vi "Lockin.Low Pass Filter Bank 2D DO NOT USE.vi"(8 "error in (no error)":errorcluster, 10 "WFms in":waveform(dbl)[][](array[waveform]), 11 "Instrument.DAQ in":refnum<class "Instrument.DAQ.lvclass">) -> (0 "error out":errorcluster, 2 "Wfms out":waveform(dbl)[][](array[waveform]), 3 "Instrument.DAQ out":refnum<class "Instrument.DAQ.lvclass">)   [LabVIEW 2019, in "Instrument.Lockin.lvlib" / "Instrument.DAQ.lvclass"]
uses:
  Instrument.DAQ.lvclass
  <vilib>/addons/Digital Filter Design/NI_DigFilterLicensed.lvlib
  <vilib>/addons/Digital Filter Design/Process.llb/DFD Filtering with State (Wfm).vi
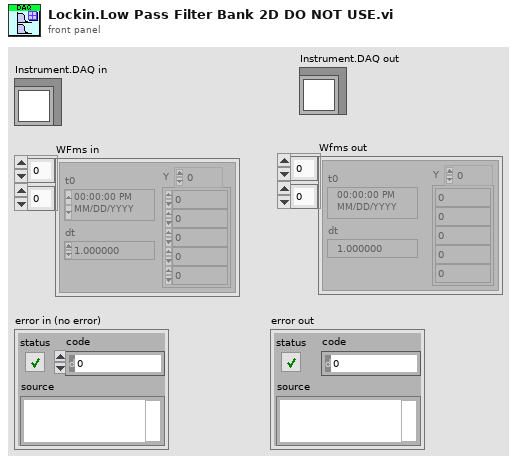
[diagram p1: front panel]
types:
  T1 = enum16{"Lowpass", "Highpass", "Bandpass", "Bandstop"}
  T2 = typedef "NI_DigFilterLicensed.lvlib/DFD Filter Obj.ctl" = cluster{"mSRate_Fs":dbl, "mSRate_Version":string, "mSRate_Comments":string, "mSRate_OrgCoef":T3, "mSRate_CurCoef":T3, "mSRate_Quantized?":bool, "mSRate_QCoef":T3, "mSRate_QSettings":T5[], "mSRate_Order":i32, "mSRate_Scaling":cluster{"mSRate_ScaleByPowerOf2?":bool, "mSRate_ScaleType":T7}}
  T3 = typedef "NI_DigFilterLicensed.lvlib/DFD Filter Coef.ctl" = cluster{"type":T4, "gain":dbl, "coef a (k)":dbl[], "coef b (v)":dbl[]}
  T4 = typedef "NI_DigFilterLicensed.lvlib/DFD Filter Structure Type Selector.ctl" = enum16{"Undefined", "FIR Direct Form", "FIR Direct Form Transposed", "FIR Symmetric", "FIR Antisymmetric", "IIR Direct Form I", "IIR Direct Form I Transposed", "IIR Direct Form II", "IIR Direct Form II Transposed", "IIR Cascaded Second Order Sections Form I", "IIR Cascaded Second Order Sections Form I Transposed", "IIR Cascaded Second Order Sections Form II", "IIR Cascaded Second Order Sections Form II Transposed", "Lattice Allpass (basic sections)", "Lattice Allpass (one multiplier sections)", "Lattice Allpass (normalized sections)", "Lattice AR (basic sections)", "Lattice AR (one multiplier sections)", "Lattice AR (normalized sections)", "Lattice MA (minimum phase)", "Lattice MA (maximum phase)", "Lattice ARMA (basic sections)", "Lattice ARMA (one multiplier sections)", "Lattice ARMA (normalized sections)"}
  T5 = typedef "NI_DigFilterLicensed.lvlib/dfd_Internal Quantization Settings.ctl" = cluster{"source":T6, "wl":i16, "iwl":i16, "overflow mode":enum16{"Saturation", "Wrap"}, "rounding mode":enum16{"Nearest", "Truncation"}, "signed?":bool}
  T6 = typedef "NI_DigFilterLicensed.lvlib/dfd_Internal Quantization Srcs.ctl" = u16
  T7 = typedef "NI_DigFilterLicensed.lvlib/DFD Coef Norm Type.ctl" = enum16{"No Norm", "Time Domain 1-Norm", "Time Domain 2-Norm", "Time Domain Inf-Norm"}
  T8 = typedef "Instrument.Lockin.lvlib/Instrument.DAQ.lvclass/REF.Channel--Cluster--Array.ctl" = T9[]
  T9 = typedef "Instrument.Lockin.lvlib/Instrument.DAQ.lvclass/REF.Channel--Cluster.ctl" = cluster{"Enable?":bool, "Channel":i32, "Frequency":dbl, "Phase":dbl, "TC":dbl, "Roll-Off":i32}
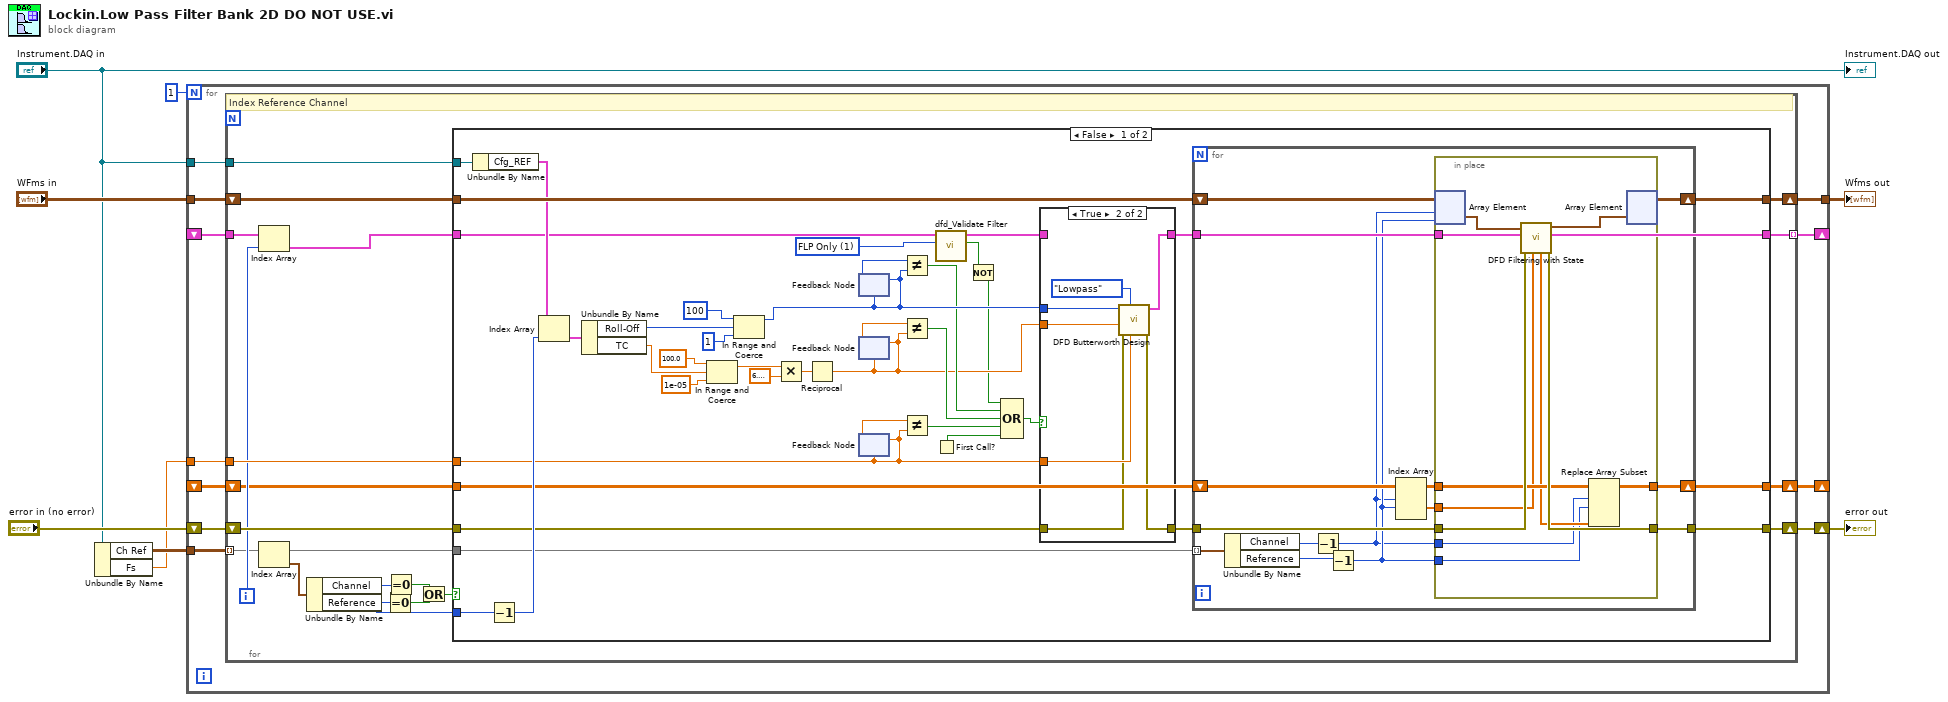
[diagram p0: block diagram]
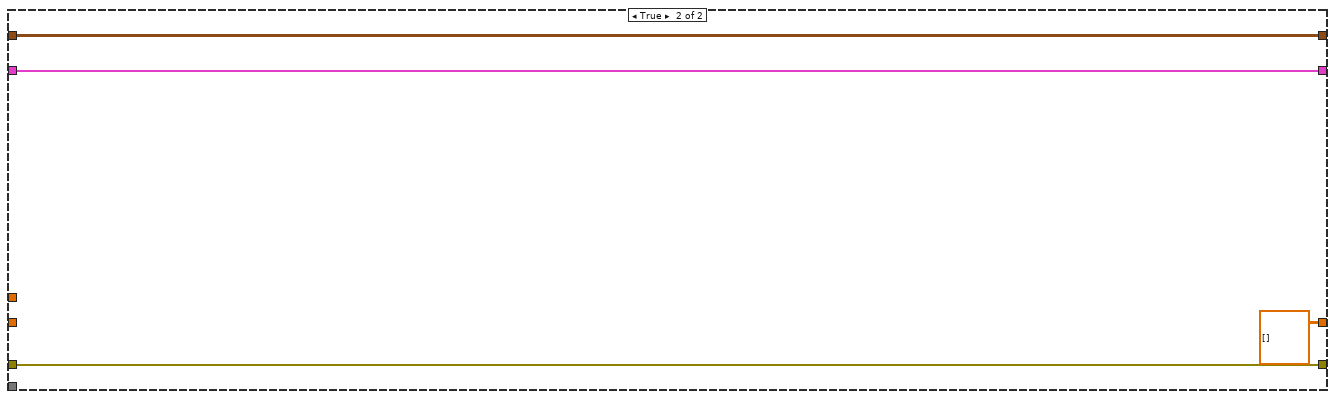
[diagram p3: hidden frame]
diagram:
  n1 = Unbundle By Name("Instrument.DAQ in") -> ("Ch Ref"=w4:cluster{"Channel":i32, "Reference":i32}[][], "Fs"=w2:dbl)
  n2 = for {
    N: 1 -> [_]
    tunnel: "WFms in" -> [w19]
    tunnel: "Instrument.DAQ in" -> [w16]
    tunnel: w4 -> [w15]
    tunnel: [w14] -> w3
    tunnel: w2 -> [w13]
    shift-right: [w18] -> w7
    shift-left: "error in (no error)" -> [w17]
    shift-right: [w11] -> _
    shift-left: _ -> [w12]
    shift-right: [w10] -> _
    shift-left: _ -> [w9]
    n3 = for {
      tunnel: w16 -> [w35]
      shift-right: [w37] -> w18
      shift-left: w17 -> [w36]
      tunnel: w15 -> [w22] mode=indexing
      tunnel: w13 -> [w28]
      tunnel: w12 -> [w25]
      tunnel: [w27] -> w11 mode=indexing
      shift-right: [w30] -> w14
      shift-left: w19 -> [w38]
      shift-right: [w21] -> w10
      shift-left: w9 -> [w20]
      i -> [w24]
      # "Index Reference Channel"
      n4 = Index Array(array=w25, index=w24) -> (element=w26:T2)
      n5 = Index Array(array=w22) -> (element=w23:cluster{"Channel":i32, "Reference":i32})  [unwired: 1 in]
      n6 = Unbundle By Name(w23) -> ("Channel"=w34:i32, "Reference"=w29:i32)
      n7 = Equal To 0?(x=w29) -> (x = 0?=w33:bool)
      n8 = Equal To 0?(x=w34) -> (x = 0?=w32:bool)
      n9 = Or(x=w32, y=w33) -> (x .or. y?=w31:bool)
      n10 = case shown="False" w31 {
        tunnel: w38 -> [w77 w114]
        tunnel: [w49 w113] -> w37
        tunnel: w36 -> [w63 w113]
        tunnel: w35 -> [w66 _]
        tunnel: [w59 w114] -> w30
        tunnel: w29 -> [w64 _]
        tunnel: w28 -> [w61 _]
        tunnel: w26 -> [w43 w112]
        tunnel: [w50 w112] -> w27
        tunnel: w22 -> [w47 _]
        tunnel: [w45 dbl[][][] []] -> w21
        tunnel: w20 -> [w44 _]
        frame False {
          w42 = u16 1 items=["Auto", "FLP Only", "FXP"] ("check option")
          n11 = Unbundle By Name(w66) -> ("Cfg_REF"=w65:T8)
          n12 = Decrement(x=w64) -> (x-1=w67:i32)
          n13 = Index Array(array=w65, index=w67) -> (element=w76:T9)
          n14 = Unbundle By Name(w76) -> ("Roll-Off"=w74:i32, "TC"=w75:dbl)
          n15 = In Range and Coerce(upper limit=100.0, x=w75, lower limit=1e-05) -> (coerced(x)=w68:dbl)  [unwired: 1 out]
          n16 = In Range and Coerce(upper limit=100, x=w74, lower limit=1) -> (coerced(x)=w60:i32)  [unwired: 1 out]
          n17 = Multiply(x=w68, y=6.283185307179586) -> (x*y=w71:dbl)
          n18 = Reciprocal(x=w71) -> (1/x=w48:dbl)
          n19 = feedback #1(w60) -> (w58:i32)
          n20 = feedback-in #1(w60) -> ()
          n21 = feedback #2(w48) -> (w56:dbl)
          n22 = feedback-in #2(w48) -> ()
          n23 = feedback #3(w61) -> (w57:dbl)
          n24 = feedback-in #3(w61) -> ()
          n25 = Not Equal?(x=w58, y=w60) -> (x != y?=w55:bool)
          n26 = Not Equal?(x=w56, y=w48) -> (x != y?=w51:bool)
          n27 = Not Equal?(x=w57, y=w61) -> (x != y?=w52:bool)
          n28 = First Call?() -> (First Call?: T/F=w54:bool)
          n29 = call <vilib>:"dfd_Validate Filter.vi"("check option"=w42, "filter in"=w43) -> ("is Valid?"=w40:bool, "filter out"=w41:T2)  [unwired: 7 in, 1 out]
          n30 = Not(x=w40) -> (.not. x?=w39:bool)
          n31 = Compound Arithmetic op=OR(w39, w55, w51, w52, w54) -> (w53:bool)
          n32 = case shown="True" w53 {
            tunnel: w61 -> [_ w110]
            tunnel: w60 -> [_ w108]
            tunnel: w48 -> [_ w107]
            tunnel: w63 -> [w103 w106]
            tunnel: [w103 w105] -> w62
            tunnel: [w102 w104] -> w50
            tunnel: w41 -> [w102 _]
            frame False {
            }
            frame True {
              n33 = call <vilib>:"DFD Butterworth Design.vi"("fs [Hz]"=w110, "filter type"=T1."Lowpass", "error in (no error)"=w106, "low cutoff freq [Hz]"=w107, "order"=w108) -> ("error out"=w105:errorcluster, "filter out"=w104:T2)  [unwired: 5 in]
            }
          }
          n34 = for {
            tunnel: w62 -> [w88]
            tunnel: w50 -> [w90]
            tunnel: [w89] -> w49
            tunnel: w47 -> [w86] mode=indexing
            shift-right: [w85] -> w59
            shift-left: w77 -> [w87]
            shift-right: [w84] -> w45
            shift-left: w44 -> [w81]
            n35 = Unbundle By Name(w86) -> ("Channel"=w82:i32, "Reference"=w83:i32)
            n36 = Decrement(x=w82) -> (x-1=w79:i32)
            n37 = Decrement(x=w83) -> (x-1=w80:i32)
            n38 = Index Array(array=w81, index (dim 0)=w79, index (dim 1)=w80) -> (element=w78:dbl[])  [unwired: 1 in]
            n39 = in-place {
              in-place-border: w90 -> [w101]
              in-place-border: [w100] -> w89
              in-place-border: w88 -> [w99]
              in-place-border: [w95] -> w84
              in-place-border: w81 -> [w96]
              in-place-border: w80 -> [w93]
              in-place-border: w79 -> [w92]
              in-place-border: w78 -> [w91]
              n40 = in-place-array #4(w87, w79, w80) -> (w98:waveform(dbl))
              n41 = call-poly <vilib>:"DFD Filtering with State.vi"("state in"=w91, "error in (no error)"=w99, "filter"=w101, "signal in"=w98) -> ("error out"=w100:errorcluster, "signal out"=w97:waveform(dbl), "state out"=w94:dbl[])  [unwired: 5 in]
              n42 = Replace Array Subset(array=w96, new element=w94, index (dim 0)=w92, index (dim 1)=w93) -> (w95:dbl[][][])  [unwired: 1 in]
              n43 = in-place-array #4(w97) -> (w85:waveform(dbl)[][])  [unwired: 2 out]
            }
          }
        }
        frame True {
        }
      }
    }
  }
  "Wfms out" <- w3
  "error out" <- w7
  "Instrument.DAQ out" <- "Instrument.DAQ in"
